vi "f_1_Qge.vi"(0 "file path (IN)":path, 1 "Project #":string, 2 "Request #":string, 3 "TEST #":string, 5 "error in (no error)":errorcluster, 6 "VGE (-ve)":dbl, 8 "VGE (+ve)":dbl) -> (11 "Di (A)":dbl, 13 "Dt (ns)":dbl, 14 "file path (OUT)":path, 15 "Qge - Delta Time (us)":dbl, 16 "Di/Dt (A/us)":dbl, 17 "DONE Qge":bool, 18 "DONE Di/Dt ON":bool, 19 "error out":errorcluster)   [LabVIEW 2020]
uses:
  Global 1.vi
  <vilib>/measure/mamon.llb/Trigger Detection for 1 Channel.vi
  <vilib>/Analysis/NI_AALBase.lvlib
  <vilib>/measure/NI_MAPro.lvlib
panel:
  out "Find Major in Histogram":dbl
  out "Histogram":dynamicdata(graph)
  out "Focus graph":waveform(dbl)(graph)
  in  "Decision ?":bool
  out "Dt (us)":dbl
  out "VGE constant point in Median Filter":dbl
  out "VGE (-ve) point":dbl
  out "Cursor a : Channel 2":dbl
  out "Cursor b : Channel 2":dbl
  out "Waveform Graph":waveform(dbl)[](graph)
  out "ON Region":waveform(dbl)[](graph) caption="Qge"
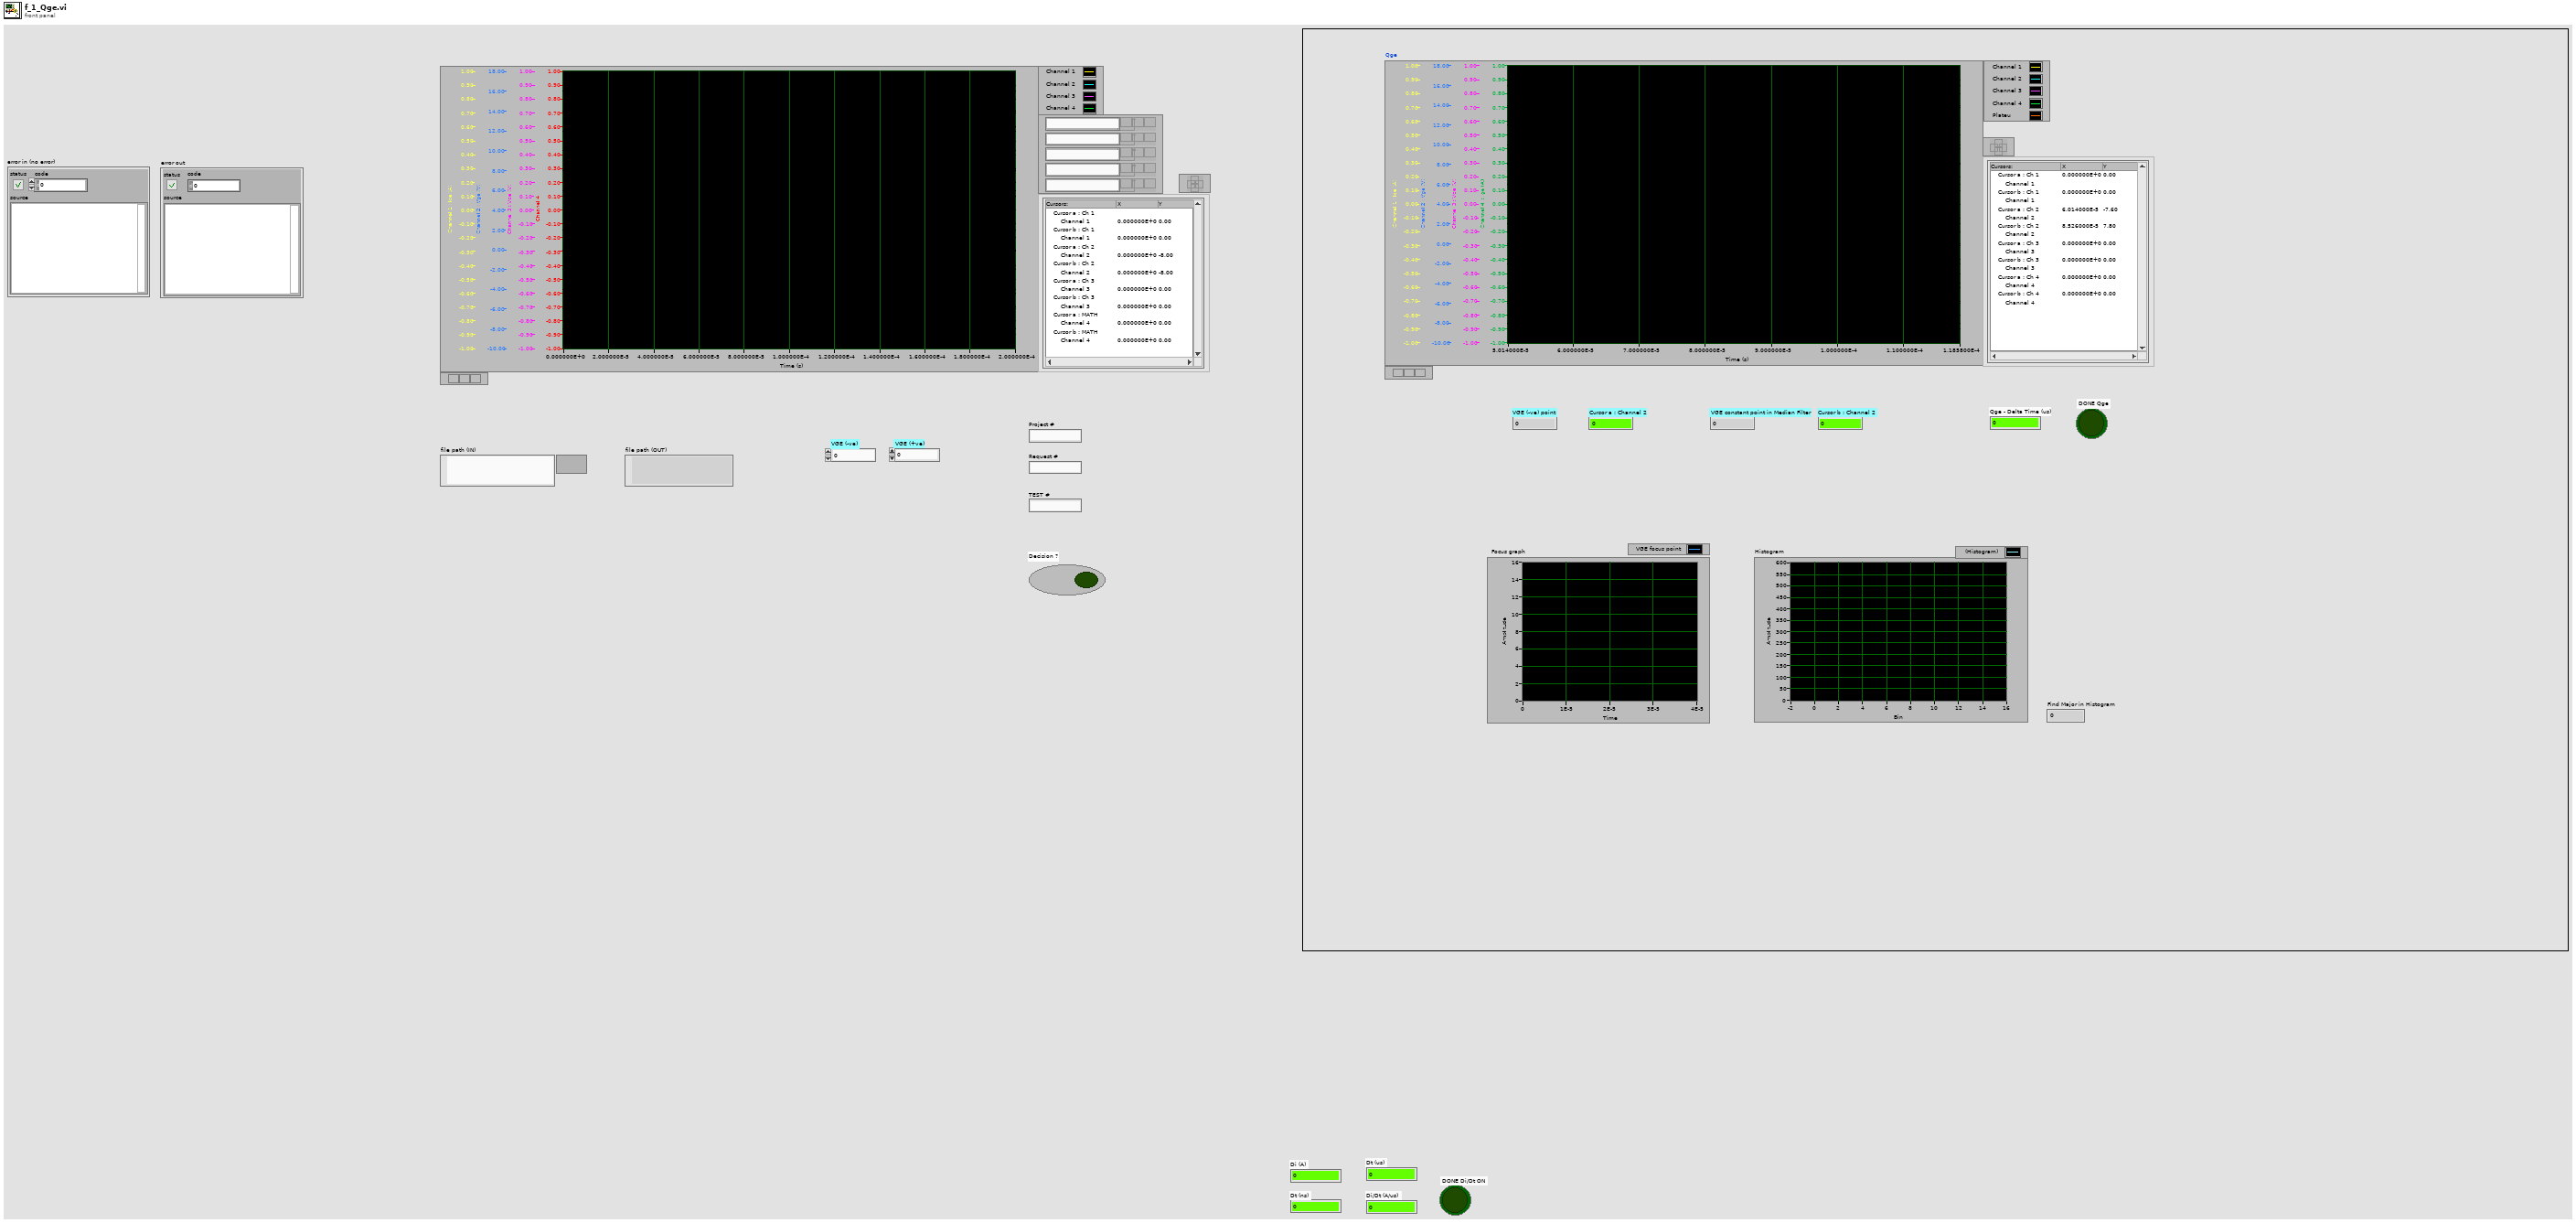
[diagram p1: front panel]
types:
  T1 = enum32{"Invalid", "Standard", "Closed", "Hidden", "Minimized", "Maximized"}
  T2 = typedef "imagedata.ctl" = cluster{"image type":i32, "image depth":i32, "image":u8[], "mask":u8[], "colors":u32[], "Rectangle":cluster{"left":i16, "top":i16, "right":i16, "bottom":i16}}
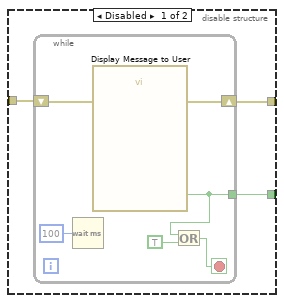
[diagram p2: hidden frame]
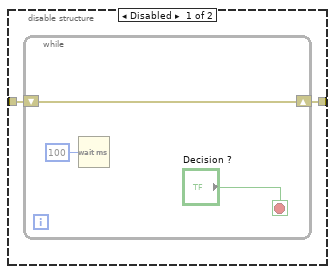
[diagram p10: hidden frame]
diagram:
  w5 = FALSE ("DONE Tdon")
  w4 = 0.0 ("Cursor a : Channel 1")
  w6 = errorcluster {"status"=FALSE, "code"=0, "source"=""} ("error out")
  w7 = waveform(dbl)[] [] ("Waveform Graph")
  n1 = local write "DONE Qge"(w5) -> ()
  n2 = local write "Cursor a : Channel 2"(w4) -> ()
  n3 = local write "Cursor b : Channel 2"(w4) -> ()
  n4 = local write "DONE Di/Dt ON"(w5) -> ()
  n5 = local write "Decision ?"(w5) -> ()
  n6 = local write "Qge - Delta Time (us)"(w4) -> ()
  n7 = local write "VGE (-ve) point"(w4) -> ()
  n8 = local write "VGE constant point in Median Filter"(w4) -> ()
  n9 = local write "Find Major in Histogram"(0.0 ("Time of Maximum")) -> ()
  n10 = local write "Di (A)"(w4) -> ()
  n11 = local write "Dt (ns)"(w4) -> ()
  n12 = local write "Dt (us)"(w4) -> ()
  n13 = local write "Di/Dt (A/us)"(w4) -> ()
  n14 = local write "error out"(w6) -> ()
  n15 = local write "error in (no error)"(w6) -> ()
  n16 = local write "Waveform Graph"(w7) -> ()
  n17 = local write "ON Region"(w7) -> ()
  n18 = local write "Histogram"(dynamicdata [] ("Histogram")) -> ()
  n19 = local write "Focus graph"(waveform(dbl) {"t0"=timestamp(0 s since 1904-01-01), "dt"=1.0, "Y"=[]} ("Focus graph")) -> ()
  n20 = flat-sequence {
    tunnel: ["file path (IN)"] -> w13
    tunnel: [w14] -> w12
    tunnel: [w23] -> w11
    tunnel: [w22] -> w10
    tunnel: w13 -> [w25]
    tunnel: w12 -> [w24]
    tunnel: [w309] -> w9
    tunnel: w11 -> [w308]
    tunnel: w10 -> [w307]
    tunnel: [w307] -> w8
    tunnel: w9 -> [w324]
    tunnel: w8 -> [w323]
    frame #0 {
      n21 = control-ref of="This VI"() -> (w19:refnum<vi>)
      n22 = invoke class="VI" method="FP.Open"(reference=w19, error in="error in (no error)", "Activate"=TRUE ("Activate?"), "State"=T1."Maximized") -> (error out=w20:errorcluster)  [unwired: 1 in, 4 out]
      n23 = property class="VI"(reference=w19, error in=w20, "Front Panel.Closeable"=TRUE ("Front Panel Window:Closeable")) -> (error out=w14:errorcluster)  [unwired: 1 out]
    }
    frame #1 {
      n24 = while {
        tunnel: w25 -> [w60]
        shift-right: [w55] -> w23
        shift-left: w24 -> [w59]
        tunnel: [w57] -> w22
        stop <- w54 stop-if-true
        n25 = flat-sequence {
          tunnel: [w90] -> w70
          tunnel: [w91] -> w69
          tunnel: w60 -> [w91]
          tunnel: w59 -> [w90]
          tunnel: w70 -> [w109]
          tunnel: w69 -> [w107]
          tunnel: [w106] -> w50
          tunnel: [w98] -> w49
          tunnel: [w92] -> w48
          tunnel: [w94] -> w47
          tunnel: [w95] -> w46
          tunnel: [w93] -> w45
          tunnel: [w96] -> w44
          tunnel: w50 -> [w149]
          tunnel: [w149] -> w43
          tunnel: w49 -> [w148]
          tunnel: [w148] -> w41
          tunnel: w48 -> [w140]
          tunnel: w47 -> [_]
          tunnel: w46 -> [w147]
          tunnel: w45 -> [w146]
          tunnel: [w146] -> w42
          tunnel: w44 -> [w145]
          tunnel: [w138] -> w40
          tunnel: [w173] -> w53
          tunnel: w43 -> [w214]
          tunnel: [w214] -> w52
          tunnel: w42 -> [w213]
          tunnel: [w213] -> w51
          tunnel: w41 -> [w169]
          tunnel: w40 -> [w162]
          tunnel: w53 -> [w227]
          tunnel: [w235] -> w39
          tunnel: w52 -> [w243]
          tunnel: [w243] -> w38
          tunnel: [w231] -> w36
          tunnel: [w234] -> w34
          tunnel: [w222] -> w32
          tunnel: [w228] -> w30
          tunnel: w51 -> [w215]
          tunnel: [w215] -> w26
          tunnel: w39 -> [w252]
          tunnel: w38 -> [w260]
          tunnel: [w260] -> w37
          tunnel: w36 -> [w259]
          tunnel: [w259] -> w35
          tunnel: w34 -> [w258]
          tunnel: [w258] -> w33
          tunnel: w32 -> [w257]
          tunnel: [w257] -> w31
          tunnel: w30 -> [w256]
          tunnel: [w256] -> w29
          tunnel: [w251] -> w28
          tunnel: [w250] -> w27
          tunnel: w26 -> [w248]
          tunnel: [w263] -> w68
          tunnel: w37 -> [w269]
          tunnel: [w269] -> w67
          tunnel: w35 -> [w268]
          tunnel: [w268] -> w66
          tunnel: w33 -> [w267]
          tunnel: [w267] -> w65
          tunnel: w31 -> [w265]
          tunnel: [w265] -> w64
          tunnel: w29 -> [w266]
          tunnel: [w266] -> w63
          tunnel: w28 -> [w264]
          tunnel: w27 -> [w262]
          tunnel: w68 -> [w281]
          tunnel: w67 -> [w293]
          tunnel: [w293] -> w62
          tunnel: w66 -> [w288]
          tunnel: w65 -> [w289]
          tunnel: w64 -> [w287]
          tunnel: w63 -> [w286]
          tunnel: [w281] -> w61
          tunnel: w62 -> [w298]
          tunnel: w61 -> [w300]
          tunnel: [w299] -> w56
          tunnel: [w298] -> w57
          frame #0 {
            w87 = waveform(dbl)[] [] ("Waveform Graph")
            w86 = 0.0 ("Cursor a : Channel 1")
            w89 = FALSE ("DONE Tdon")
            n26 = local write "DONE Qge"(w89) -> ()
            n27 = local write "VGE (-ve) point"(w86) -> ()
            n28 = local write "Cursor a : Channel 2"(w86) -> ()
            n29 = local write "Cursor b : Channel 2"(w86) -> ()
            n30 = local write "DONE Di/Dt ON"(w89) -> ()
            n31 = local write "Decision ?"(w89) -> ()
            n32 = local write "Di (A)"(w86) -> ()
            n33 = local write "Dt (ns)"(w86) -> ()
            n34 = local write "Dt (us)"(w86) -> ()
            n35 = local write "Di/Dt (A/us)"(w86) -> ()
            n36 = local write "VGE constant point in Median Filter"(w86) -> ()
            n37 = local write "Qge - Delta Time (us)"(w86) -> ()
            n38 = Wait (ms)(milliseconds to wait=u32 200) -> ()  [unwired: 1 out]
            n39 = Wait (ms)(milliseconds to wait=u32 200) -> ()  [unwired: 1 out]
            n40 = local write "Find Major in Histogram"(0.0 ("Time of Maximum")) -> ()
            n41 = local write "Histogram"(dynamicdata [] ("Histogram")) -> ()
            n42 = local write "ON Region"(w87) -> ()
            n43 = local write "Waveform Graph"(w87) -> ()
            n44 = local write "Focus graph"(waveform(dbl) {"t0"=timestamp(0 s since 1904-01-01), "dt"=1.0, "Y"=[]} ("Focus graph")) -> ()
          }
          frame #1 {
            w98 = 0.0 ("number")
            # "Channel 2"
            # "Channel 4"
            # "t0"
            # "Channel 1"
            # "Channel 3"
            # "dt"
            # "Ch1"
            n45 = call "3_ReadDatatoWaveform.vi"("file path (IN)"=w107, "error in (no error)"=w109) -> ("Ch 1 Data"=w105:dbl[], "Ch 2 Data"=w100:dbl[], "file path (OUT)"=w106:path, "Waveform Graph"=→"Waveform Graph":waveform(dbl)[], "Ch 3 Data"=w104:dbl[], "Ch 4 Data"=w102:dbl[], "dt"=w95:dbl, "error out"=w108:errorcluster)  [unwired: 5 in, 1 out]
            n46 = To Time Stamp(1:w98) -> (0:w101:timestamp)
            n47 = disable-structure shown="Enabled" {
              disable-tunnel: w101 -> [w125 _]
              disable-tunnel: w95 -> [w124 _]
              disable-tunnel: w100 -> [w123 _]
              disable-tunnel: [w122 _] -> w94
              frame Enabled {
                # "Channel 2"
                n48 = Bundle By Name("Y"=w123, "dt"=w124, "t0"=w125) -> (w122:waveform(dbl))  [unwired: 1 in]
              }
              frame Disabled {
              }
            }
            n49 = disable-structure shown="Enabled" {
              disable-tunnel: w101 -> [w137 _]
              disable-tunnel: w95 -> [w136 _]
              disable-tunnel: w104 -> [w135 _]
              disable-tunnel: [w134 _] -> w110
              frame Enabled {
                # "Channel 3"
                n50 = Bundle By Name("Y"=w135, "dt"=w136, "t0"=w137) -> (w134:waveform(dbl))  [unwired: 1 in]
              }
              frame Disabled {
              }
            }
            n51 = disable-structure shown="Enabled" {
              disable-tunnel: w101 -> [w129 _]
              disable-tunnel: w95 -> [w128 _]
              disable-tunnel: w102 -> [w127 _]
              disable-tunnel: [w126 _] -> w97
              frame Enabled {
                # "Channel 4"
                n52 = Bundle By Name("Y"=w127, "dt"=w128, "t0"=w129) -> (w126:waveform(dbl))  [unwired: 1 in]
              }
              frame Disabled {
              }
            }
            n53 = disable-structure shown="Enabled" {
              disable-tunnel: w101 -> [w133 _]
              disable-tunnel: w95 -> [w132 _]
              disable-tunnel: w105 -> [w131 _]
              disable-tunnel: [w130 _] -> w111
              frame Enabled {
                # "Channel 1"
                n54 = Bundle By Name("Y"=w131, "dt"=w132, "t0"=w133) -> (w130:waveform(dbl))  [unwired: 1 in]
              }
              frame Disabled {
              }
            }
            n55 = property on="Waveform Graph" class="WFGraph (strict)"(error in=w108, "XScale.Offset"=w98) -> (error out=w92:errorcluster)  [unwired: 1 in, 1 out]
            n56 = disable-structure shown="Enabled" {
              disable-tunnel: w94 -> [w120 _]
              disable-tunnel: [w119 _] -> w93
              disable-tunnel: [w118 _] -> w96
              disable-tunnel: w95 -> [w117 _]
              frame Enabled {
                # "OG = 30"
                # "Median"
                n57 = global read "Global 1.vi" "Median Filter Rank"() -> (w116:i32)
                n58 = Unbundle By Name(w120) -> ("Y"=w121:dbl[])
                n59 = call <vilib>:"Median Filter.vi"("right rank"=w116, "left rank"=w116, "X"=w121) -> ("Filtered X"=w118:dbl[])  [unwired: 7 in, 1 out]
                n60 = Bundle By Name("Y"=w118, "dt"=w117) -> (w119:waveform(dbl))  [unwired: 1 in]
              }
              frame Disabled {
              }
            }
            n61 = Build Array(w111, w94, w110, w97, w93) -> (→"ON Region":waveform(dbl)[])
            n62 = Wait (ms)(milliseconds to wait=u32 200) -> ()  [unwired: 1 out]
            n63 = call <vilib>:"Beep.vi"("use system alert? (T)"=FALSE, "duration (msec)"=u32 200, "frequency (Hz)"=u32 2000) -> ()  [unwired: 9 in]
          }
          frame #2 {
            n64 = disable-structure shown="Enabled" {
              disable-tunnel: w147 -> [_ w155]
              disable-tunnel: w145 -> [_ w151]
              disable-tunnel: [_ w150] -> w143
              frame Disabled {
              }
              frame Enabled {
                # "Remains"
                # "Find (+ve)"
                # "Find 0"
                n65 = Search 1D Array(1D array=w151, element=0.0, start index (0)=0) -> (index of element=w156:i32)
                n66 = Split 1D Array(array=w151, index=w156) -> (second subarray=w159:dbl[])  [unwired: 1 out]
                n67 = Search 1D Array(1D array=w159, element="VGE (+ve)", start index (0)=0) -> (index of element=w158:i32)
                n68 = Split 1D Array(array=w159, index=w158) -> (first subarray=w160:dbl[])  [unwired: 1 out]
                n69 = Bundle By Name("Y"=w160, "dt"=w155) -> (w150:waveform(dbl))  [unwired: 1 in]
                "Focus graph" <- w150
              }
            }
            n70 = Wait (ms)(milliseconds to wait=u32 200) -> ()  [unwired: 1 out]
            n71 = call "Create Histogram"("error in (no error)"=w140, "Signal"=w143) -> ("error out"=w139:errorcluster, "Histogram"=w142:dynamicdata)  [unwired: 8 in]
            "Histogram" <- w142
            n72 = call "Statistics"("Signals"=w142, "error in (no error)"=w139) -> ("Time of Maximum"=→"Find Major in Histogram":dynamicdata, "error out"=w138:errorcluster)  [unwired: 24 in]
          }
          frame #3 {
            n73 = property on="ON Region" class="WFGraph (strict)"(error in=w162) -> (error out=w170:errorcluster, "Width"=w171:u32)  [unwired: 1 in, 1 out]
            n74 = property on="ON Region" class="WFGraph (strict)"(error in=w170, "Caption.Justify"=enum16{"Left", "Center", "Right"}."Left" ("Caption.Justification"), "Caption.Width"=w171, "Caption.FontBold"=TRUE ("Caption.Font:Bold"), "Caption.FontColor"=u32 16860 ("Caption.Font:Color"), "Caption.FontSize"=u32 24 ("Caption.Font:Size"), "Caption.Text"="Qge") -> (error out=w172:errorcluster)  [unwired: 1 in, 1 out]
            n75 = Wait (ms)(milliseconds to wait=u32 200) -> ()  [unwired: 1 out]
            n76 = property on="ON Region" class="WFGraph (strict)"(error in=w172, "XScale.Offset"=w169) -> (error out=w163:errorcluster)  [unwired: 1 in, 1 out]
            n77 = property on="ON Region" class="WFGraph (strict)"(error in=w163, "Active Cursor"=u32 0, "Cursor.Cursor X"=0.0 ("Cursor.Cursor Position:Cursor X"), "Cursor.Cursor Y"=0.0 ("Cursor.Cursor Position:Cursor Y"), "Cursor.Visible"=FALSE) -> (error out=w206:errorcluster)  [unwired: 1 in, 1 out]
            n78 = property on="ON Region" class="WFGraph (strict)"(error in=w206, "Active Cursor"=u32 1, "Cursor.Cursor X"=0.0 ("Cursor.Cursor Position:Cursor X"), "Cursor.Cursor Y"=0.0 ("Cursor.Cursor Position:Cursor Y"), "Cursor.Visible"=FALSE) -> (error out=w207:errorcluster)  [unwired: 1 in, 1 out]
            n79 = property on="ON Region" class="WFGraph (strict)"(error in=w207, "Active Cursor"=u32 2, "Cursor.Cursor X"=0.0 ("Cursor.Cursor Position:Cursor X"), "Cursor.Cursor Y"=0.0 ("Cursor.Cursor Position:Cursor Y"), "Cursor.Visible"=FALSE) -> (error out=w208:errorcluster)  [unwired: 1 in, 1 out]
            n80 = property on="ON Region" class="WFGraph (strict)"(error in=w208, "Active Cursor"=u32 3, "Cursor.Cursor X"=0.0 ("Cursor.Cursor Position:Cursor X"), "Cursor.Cursor Y"=0.0 ("Cursor.Cursor Position:Cursor Y"), "Cursor.Visible"=FALSE) -> (error out=w209:errorcluster)  [unwired: 1 in, 1 out]
            n81 = property on="ON Region" class="WFGraph (strict)"(error in=w209, "Active Cursor"=u32 4, "Cursor.Cursor X"=0.0 ("Cursor.Cursor Position:Cursor X"), "Cursor.Cursor Y"=0.0 ("Cursor.Cursor Position:Cursor Y"), "Cursor.Visible"=FALSE) -> (error out=w210:errorcluster)  [unwired: 1 in, 1 out]
            n82 = property on="ON Region" class="WFGraph (strict)"(error in=w210, "Active Cursor"=u32 5, "Cursor.Cursor X"=0.0 ("Cursor.Cursor Position:Cursor X"), "Cursor.Cursor Y"=0.0 ("Cursor.Cursor Position:Cursor Y"), "Cursor.Visible"=FALSE) -> (error out=w211:errorcluster)  [unwired: 1 in, 1 out]
            n83 = property on="ON Region" class="WFGraph (strict)"(error in=w211, "Active Cursor"=u32 6, "Cursor.Cursor X"=0.0 ("Cursor.Cursor Position:Cursor X"), "Cursor.Cursor Y"=0.0 ("Cursor.Cursor Position:Cursor Y"), "Cursor.Visible"=FALSE) -> (error out=w212:errorcluster)  [unwired: 1 in, 1 out]
            n84 = property on="ON Region" class="WFGraph (strict)"(error in=w212, "Active Cursor"=u32 7, "Cursor.Cursor X"=0.0 ("Cursor.Cursor Position:Cursor X"), "Cursor.Cursor Y"=0.0 ("Cursor.Cursor Position:Cursor Y"), "Cursor.Visible"=FALSE) -> (error out=w173:errorcluster)  [unwired: 1 in, 1 out]
          }
          frame #4 {
            w224 = u16 1 items=["Falling Edge", "Rising Edge"] ("trigger slope")
            w225 = u16 1 items=["Index", "Time"] ("location mode")
            w229 = u16 1 items=["Falling Edge", "Rising Edge"] ("trigger slope")
            w230 = u16 1 items=["Index", "Time"] ("location mode")
            # "Cursor a : Channel 1"
            # "Cursor b : Channel 1"
            # "Cursor b : Channel 1"
            # "Cursor a : Channel 1"
            # "Cursor b : Channel 1"
            # "Cursor a : Channel 1"
            # "Cursor b : Channel 1"
            # "Cursor a : Channel 1"
            # "End Time 1st Cursor"
            # "End Time 2nd Cursor"
            # "1st PARAMETER : VGE (-ve)"
            # "Channel 2"
            # "2nd PARAMETER : VGE constant point"
            # "Channel 2"
            n85 = Add(x="VGE (-ve)", y=0.3) -> (x+y=w218:dbl)
            n86 = call-poly <vilib>:"Basic Level Trigger Detection.vi"("signal in"=w215, "level"=w218, "location mode"=w230, "error in (no error)"=w227, "trigger slope"=w229) -> ("trigger location"=w228:dbl, "error out"=w226:errorcluster)  [unwired: 8 in, 1 out]
            n87 = property on="ON Region" class="WFGraph (strict)"(error in=w226, "Active Cursor"=u32 2, "Cursor.Cursor X"=w228, "Cursor.Visible"=TRUE, "Cursor.Cursor Name Visible"=TRUE) -> (error out=w239:errorcluster)  [unwired: 1 in, 1 out]
            n88 = property on="ON Region" class="WFGraph (strict)"(error in=w239, "Active Cursor"=u32 2) -> (error out=w221:errorcluster, "Cursor.Cursor Y"=w231:dbl)  [unwired: 1 in, 1 out]
            "Cursor a : Channel 2" <- w231
            n89 = local read "Find Major in Histogram"() -> (w220:dbl)
            "VGE constant point in Median Filter" <- w220
            n90 = call-poly <vilib>:"Basic Level Trigger Detection.vi"("signal in"=w215, "level"=w220, "location mode"=w225, "error in (no error)"=w221, "trigger slope"=w224) -> ("trigger location"=w222:dbl, "error out"=w223:errorcluster)  [unwired: 8 in, 1 out]
            n91 = Wait (ms)(milliseconds to wait=u32 200) -> ()  [unwired: 1 out]
            n92 = property on="ON Region" class="WFGraph (strict)"(error in=w223, "Active Cursor"=u32 3, "Cursor.Cursor X"=w222, "Cursor.Visible"=TRUE, "Cursor.Cursor Name Visible"=TRUE) -> (error out=w236:errorcluster)  [unwired: 1 in, 1 out]
            n93 = call <vilib>:"Beep.vi"("use system alert? (T)"=FALSE, "duration (msec)"=u32 200, "frequency (Hz)"=u32 2000) -> ()  [unwired: 9 in]
            n94 = property on="ON Region" class="WFGraph (strict)"(error in=w236, "Active Cursor"=u32 3) -> (error out=w235:errorcluster, "Cursor.Cursor Y"=w234:dbl)  [unwired: 1 in, 1 out]
            "Cursor b : Channel 2" <- w234
            "VGE (-ve) point" <- "VGE (-ve)"
          }
          frame #5 {
            w254 = u16 1 items=["Falling Edge", "Rising Edge"] ("trigger slope")
            w253 = u16 1 items=["Index", "Time"] ("location mode")
            # "VGE +ve"
            # "Channel 2"
            n95 = local read "VGE (+ve)"() -> (w255:dbl)
            n96 = call-poly <vilib>:"Basic Level Trigger Detection.vi"("signal in"=w248, "level"=w255, "location mode"=w253, "error in (no error)"=w252, "trigger slope"=w254) -> ("trigger location"=w250:dbl, "error out"=w251:errorcluster)  [unwired: 8 in, 1 out]
            n97 = Wait (ms)(milliseconds to wait=u32 200) -> ()  [unwired: 1 out]
          }
          frame #6 {
            n98 = disable-structure shown="Enabled" {
              disable-tunnel: w264 -> [w277 w278]
              disable-tunnel: [w276 w278] -> w263
              disable-tunnel: w266 -> [w271 _]
              disable-tunnel: w262 -> [w270 _]
              frame Enabled {
                # "2nd Cursor"
                # "1st Cursor"
                n99 = Subtract(x=w271, y=1e-05) -> (x-y=w272:dbl)
                n100 = Add(x=w270, y=1e-05) -> (x+y=w273:dbl)
                n101 = property on="ON Region" class="WFGraph (strict)"(error in=w277, "XScale.Minimum"=w272, "XScale.Maximum"=w273) -> (error out=w276:errorcluster)  [unwired: 1 in, 1 out]
              }
              frame Disabled {
              }
            }
            n102 = Wait (ms)(milliseconds to wait=u32 200) -> ()  [unwired: 1 out]
          }
          frame #7 {
            # "us"
            # "ns"
            n103 = Subtract(x=w289, y=w288) -> (x-y=w284:dbl)
            n104 = Subtract(x=w287, y=w286) -> (x-y=w285:dbl)
            n105 = Absolute Value(x=w284) -> (abs(x)=w283:dbl)
            "Di (A)" <- w283
            n106 = Absolute Value(x=w285) -> (abs(x)=w282:dbl)
            n107 = Multiply(x=w282, y=1000000000.0) -> (x*y=→"Dt (ns)":dbl)
            n108 = Multiply(x=w282, y=1000000.0) -> (x*y=w279:dbl)
            "Qge - Delta Time (us)" <- w279
            "Dt (us)" <- w279
            n109 = call <vilib>:"Beep.vi"("use system alert? (T)"=FALSE, "duration (msec)"=u32 200, "frequency (Hz)"=u32 2000) -> ()  [unwired: 9 in]
            n110 = Wait (ms)(milliseconds to wait=u32 200) -> ()  [unwired: 1 out]
            n111 = Divide(x=w283, y=w279) -> (x/y=→"Di/Dt (A/us)":dbl)
          }
          frame #8 {
            n112 = disable-structure shown="Enabled" {
              disable-tunnel: w300 -> [w302 w306]
              disable-tunnel: [w301 w306] -> w299
              frame Disabled {
                n113 = while {
                  shift-right: [w303] -> w301
                  shift-left: w302 -> [w303]
                  stop <- "Decision ?" stop-if-true
                  n114 = Wait (ms)(milliseconds to wait=u32 100) -> ()  [unwired: 1 out]
                }
              }
              frame Enabled {
              }
            }
          }
        }
        n115 = disable-structure shown="Enabled" {
          disable-tunnel: w56 -> [w73 w80]
          disable-tunnel: [w72 w80] -> w55
          disable-tunnel: [w71 TRUE ("NO")] -> w54
          frame Disabled {
            n116 = while {
              tunnel: [w75] -> w71
              shift-right: [w78] -> w72
              shift-left: w73 -> [w79]
              stop <- w77 stop-if-true
              n117 = Wait (ms)(milliseconds to wait=u32 100) -> ()  [unwired: 1 out]
              n118 = call "Display Message to User"("error in (no error)"=w79) -> ("error out"=w78:errorcluster, "NO"=w75:bool)  [unwired: 9 in]
              n119 = Or(x=w75, y=TRUE) -> (x .or. y?=w77:bool)
            }
          }
          frame Enabled {
          }
        }
        n120 = Wait (ms)(milliseconds to wait=u32 100) -> ()  [unwired: 1 out]
      }
    }
    frame #2 {
      w312 = "_"
      n121 = invoke on="ON Region" class="WFGraph (strict)" method="Get Image"(error in=w308) -> (error out=w316:errorcluster, "image data"=w319:T2)  [unwired: 5 in, 4 out]
      n122 = Concatenate Strings("C:\\GateCharge_Project\\GateCharge_Image\\" ("string"), "Project #", w312, "Request #", w312, "TEST #", w312, "Qge" ("string"), ".png" ("string")) -> (w320:string)
      n123 = String To Path(string=w320) -> (path=w318:path)
      n124 = call <vilib>:"Write PNG File.vi"("error in (no error)"=w316, "image data"=w319, "path to PNG file"=w318) -> ("error out"=w309:errorcluster)  [unwired: 7 in, 1 out]
      "DONE Qge" <- TRUE ("DONE Tdon")
      "DONE Di/Dt ON" <- TRUE ("DONE Di/Dt ON")
    }
    frame #3 {
      n125 = disable-structure shown="Enabled" {
        disable-tunnel: w324 -> [w325 _]
        frame Enabled {
          n126 = control-ref of="This VI"() -> (w326:refnum<vi>)
          n127 = invoke class="VI" method="FP.Close"(reference=w326, error in=w325) -> ()  [unwired: 1 in, 3 out]
        }
        frame Disabled {
        }
      }
      "error out" <- w324
      "file path (OUT)" <- w323
    }
  }
